vi "Valid Syntax List.vi"(0 "functionbase in":refnum<class "functionbase.lvclass">, 11 "error in (no error)":errorcluster) -> (4 "functionbase out":refnum<class "functionbase.lvclass">, 6 "Syntax List":T1[](array[typedef]), 15 "error out":errorcluster)   [LabVIEW 2016, in "functionbase.lvclass"]
uses:
  functionbase.lvclass
  common/Syntax Format.ctl
  common/Variable#.ctl
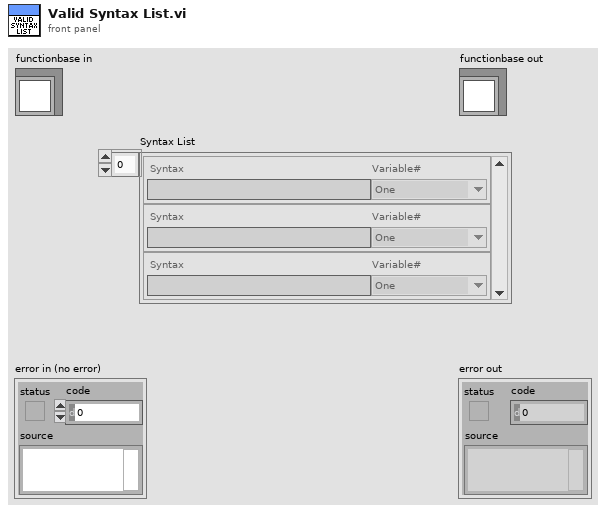
[diagram p1: front panel]
types:
  T1 = typedef "Syntax Format.ctl" = cluster{"Syntax":string, "Variable#":T2}
  T2 = typedef "Variable#.ctl" = enum16{"Zero", "One", "Two", "Three", "Four", "Five"}
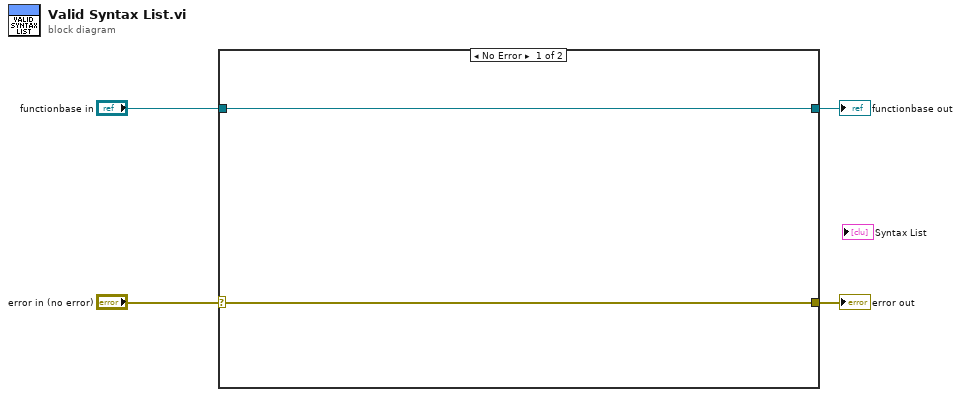
[diagram p0: block diagram]
diagram:
  n1 = case shown="No Error" "error in (no error)" {
    selector: "error in (no error)" -> [w5 w8]
    tunnel: [w5 w8] -> w3
    tunnel: [w6 w7] -> w1
    tunnel: "functionbase in" -> [w6 w7]
    frame No Error {
    }
    frame Error {
    }
  }
  "error out" <- w3
  "functionbase out" <- w1
